vi "Interpret Licor Parameter-String.vi"(7 "Tabellen-String":string) -> (8 "Parameter":dbl[](array[numeric]))   [LabVIEW 2010, in "LicorLI7000.lvlib"]
uses:
  LicorLI7000.lvlib
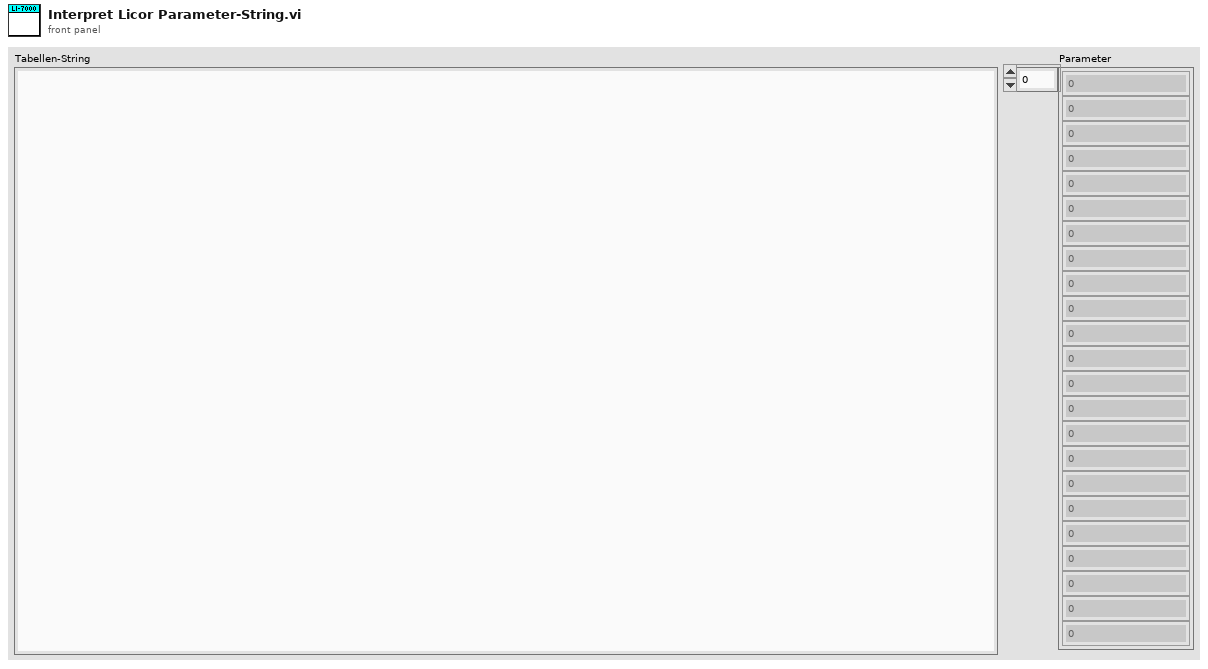
[diagram p1: front panel]
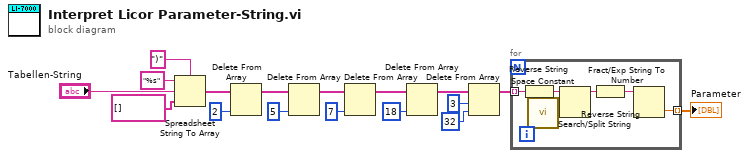
[diagram p0: block diagram]
diagram:
  n1 = Spreadsheet String To Array(delimiter (Tab)=")" ("Trennzeichen (Tabulator)"), format string="%s" ("Format-String"), spreadsheet string="Tabellen-String", array type (2D Dbl)=string[] []) -> (array=w13:string[])
  n2 = Delete From Array(array=w13, index=2 ("Länge")) -> (array with subset deleted=w4:string[])  [unwired: 1 in, 1 out]
  n3 = Delete From Array(array=w4, index=5 ("Länge")) -> (array with subset deleted=w5:string[])  [unwired: 1 in, 1 out]
  n4 = Delete From Array(array=w5, index=7 ("Länge")) -> (array with subset deleted=w6:string[])  [unwired: 1 in, 1 out]
  n5 = Delete From Array(array=w6, index=18 ("Länge")) -> (array with subset deleted=w7:string[])  [unwired: 1 in, 1 out]
  n6 = Delete From Array(array=w7, length=3 ("Index"), index=32 ("Länge")) -> (array with subset deleted=w15:string[])  [unwired: 1 out]
  n7 = for {
    tunnel: w15 -> [w21] mode=indexing
    tunnel: [w22] -> w17 mode=indexing
    n8 = Reverse String(1:w21) -> (0:w20:string)
    n9 = call <vilib>:"Space Constant.vi"() -> ("String"=w23:string)
    n10 = Search/Split String(string=w20, search string/char (-)=w23) -> (substring before match=w19:string)  [unwired: 1 in, 2 out]
    n11 = Reverse String(1:w19) -> (0:w18:string)
    n12 = Fract/Exp String To Number(string=w18) -> (number=w22:dbl)  [unwired: 3 in, 1 out]
  }
  "Parameter" <- w17
